vi "Hello.vi"(0 "MAC Address in Hex":string, 5 "error in (no error)":errorcluster) -> (6 "Reset to factory Frame":string, 8 "error out":errorcluster)   [LabVIEW 2015]
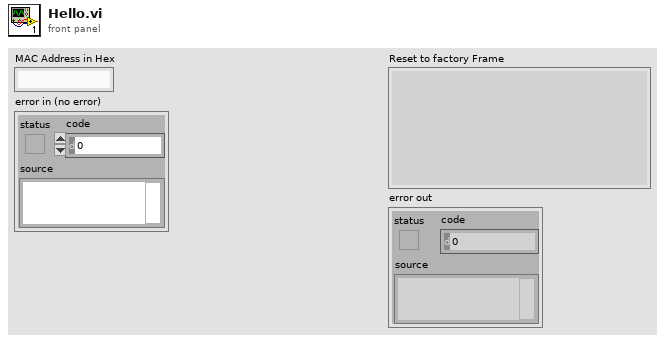
[diagram p1: front panel]
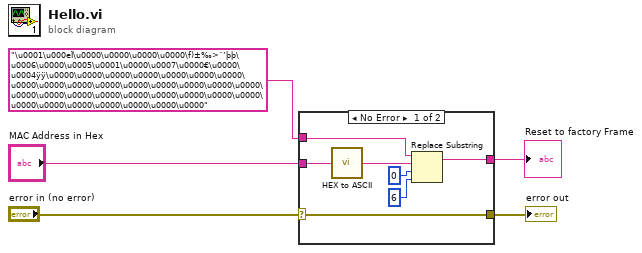
[diagram p0: block diagram]
diagram:
  n1 = case shown="No Error" "error in (no error)" {
    selector: "error in (no error)" -> [w6 w13]
    tunnel: "\u0001\u000eÏ\u0000\u0000\u0000\u0000\f)±‰>ˆ’þþ\u0006\u0000\u0005\u0001\u0000\u0007\u0000€\u0000\u0004ÿÿ\u0000\u0000\u0000\u0000\u0000\u0000\u0000\u0000\u0000\u0000\u0000\u0000\u0000\u0000\u0000\u0000\u0000\u0000\u0000\u0000\u0000\u0000\u0000\u0000\u0000\u0000\u0000\u0000\u0000\u0000\u0000\u0000" -> [w9 _]
    tunnel: "MAC Address in Hex" -> [w8 _]
    tunnel: [w7 _] -> w3
    tunnel: [w6 w13] -> w1
    frame No Error {
      n2 = call "HEX to ASCII.vi"("String in HEX"=w8) -> ("String in ASCII"=w11:string)
      n3 = Replace Substring(2:6 ("offset (0)"), 3:0 ("length (len. of substring)"), 4:w11, 5:w9) -> (1:w7:string)  [unwired: 1 out]
    }
    frame Error {
    }
  }
  "Reset to factory Frame" <- w3
  "error out" <- w1
